vi "InBoundsCheck.vi"(10 "Stats in":dbl[][](array[numeric]), 11 "RawVmagUVWCone in":dbl[](array[numeric])) -> (0 "allGood":bool)   [LabVIEW 2016]
panel:
  out "In Range?":bool[](array[boolean])
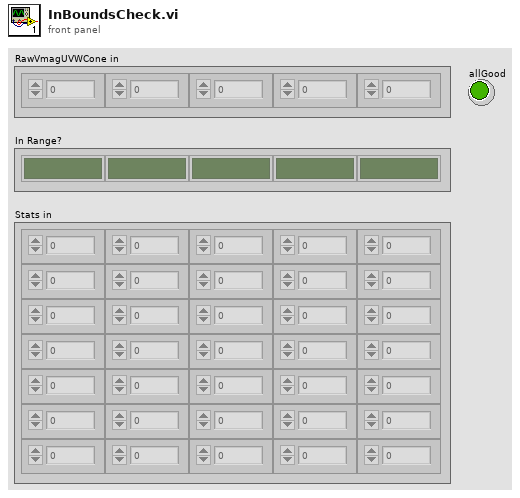
[diagram p1: front panel]
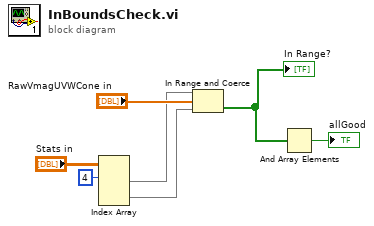
[diagram p0: block diagram]
diagram:
  n1 = Index Array(array="Stats in", index (row) #1=4 ("index (row)")) -> (element #1=w4:dbl[], element #2=w3:dbl[])  [unwired: 3 in]
  n2 = In Range and Coerce(upper limit=w4, x="RawVmagUVWCone in", lower limit=w3) -> (In Range?=w2:bool[])  [unwired: 1 out]
  "In Range?" <- w2
  n3 = And Array Elements(Boolean array=w2) -> (logical AND=→"allGood":bool)
